vi "DSG Generate Waveform.vi"(6 "hardware commands sync queue":T2, 7 "measurement configuration":T1={"Input channel"=0, "Full scale range"=10.0, "Analog source resource name"="", "Frequency"=1000.0, "Amplitude"=-1.0, "Digital capture resource name"="", "Digital capture sample rate"=800000.0, "Digital capture samples"=800000}, 8 "error in":errorcluster, 10 "DAQmx product name":string, 11 "DSG task in":refnum<k21>) -> (0 "error out":errorcluster, 3 "DSG task out":refnum<k21>)   [LabVIEW 2021, in "AC_ADC.lvlib"]
uses:
  AC_ADC.lvlib
  shared/subVIs/controls/HW Sync Commands Queue Ref.ctl
  shared/subVIs/controls/HW Sync Commands.ctl
  Measurement Configuration.ctl
  <vilib>/addons/_NISVFA/_Generation/Signal Generation/SV Signal/sv_System Timing Model.ctl
  <vilib>/DAQmx/write.llb/DAQmx Write (Analog 1D Wfm NChan NSamp).vi
  <vilib>/addons/_NISVFA/_Generation/Signal Generation/SV Sinusoid/SV Sinusoid.lvclass
  C:/Program Files/National Instruments/LabVIEW 2021/vi.lib/addons/_NISVFA/_Generation/Signal Generation/SV Signal/SV Signal.lvclass
  <vilib>/addons/_NISVFA/_Generation/Signal Generation/SV Sinusoid/Configure Sine.vi
  <vilib>/addons/_NISVFA/_Generation/Signal Generation/SV Signal/Write Sample Rate.vi
  <vilib>/addons/_NISVFA/_Generation/Signal Generation/SV Signal/Write System Timing Model.vi
  <vilib>/addons/_NISVFA/_Generation/Signal Generation/SV Signal/Write Ramp Parameters.vi
  <vilib>/DAQmx/miscellaneous.llb/DAQmx Fill In Error Info.vi
  <resource>/objmgr/daqmx.rc
  <vilib>/addons/_NISVFA/_Generation/Signal Generation/SV Signal/SV Signal.lvclass
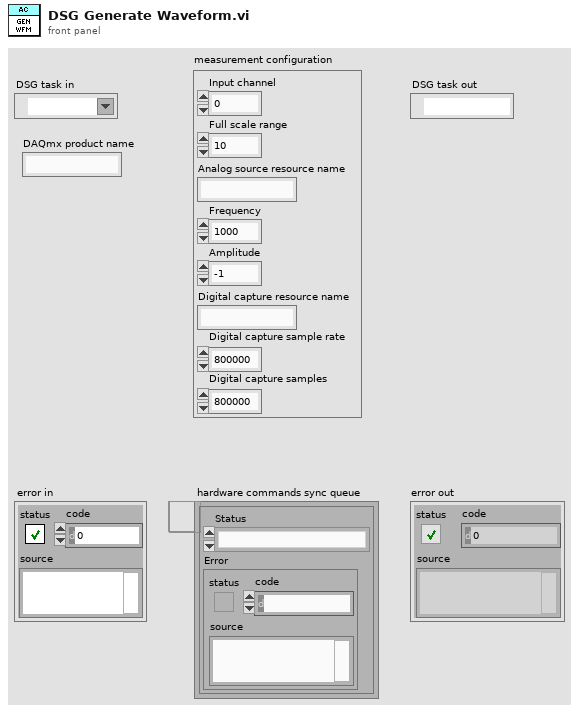
[diagram p1: front panel]
types:
  T1 = typedef "AC_ADC.lvlib/Measurement Configuration.ctl" = cluster{"Input channel":i32, "Full scale range":dbl, "Analog source resource name":string, "Frequency":dbl, "Amplitude":dbl, "Digital capture resource name":string, "Digital capture sample rate":dbl, "Digital capture samples":u32}
  T2 = typedef "HW Sync Commands Queue Ref.ctl" = refnum<queue>
  T3 = enum16{"NoAction", "GenerationStarted", "AcquisitionCompleted", "GenerationErrored"}
  T4 = cluster{"profile":enum16{"Linear", "Half cosine"}, "durations [s]":cluster{"ramp-up":dbl, "transition":dbl, "ramp-down":dbl}}
  T5 = typedef "HW Sync Commands.ctl" = enum16{"NoAction", "GenerationStarted", "AcquisitionCompleted", "GenerationErrored"}
  T6 = cluster{"element":enum16{"NoAction", "GenerationStarted", "AcquisitionCompleted", "GenerationErrored"}, "error out":errorcluster}
  T7 = typedef "SV Signal.lvclass/sv_System Timing Model.ctl" = i64
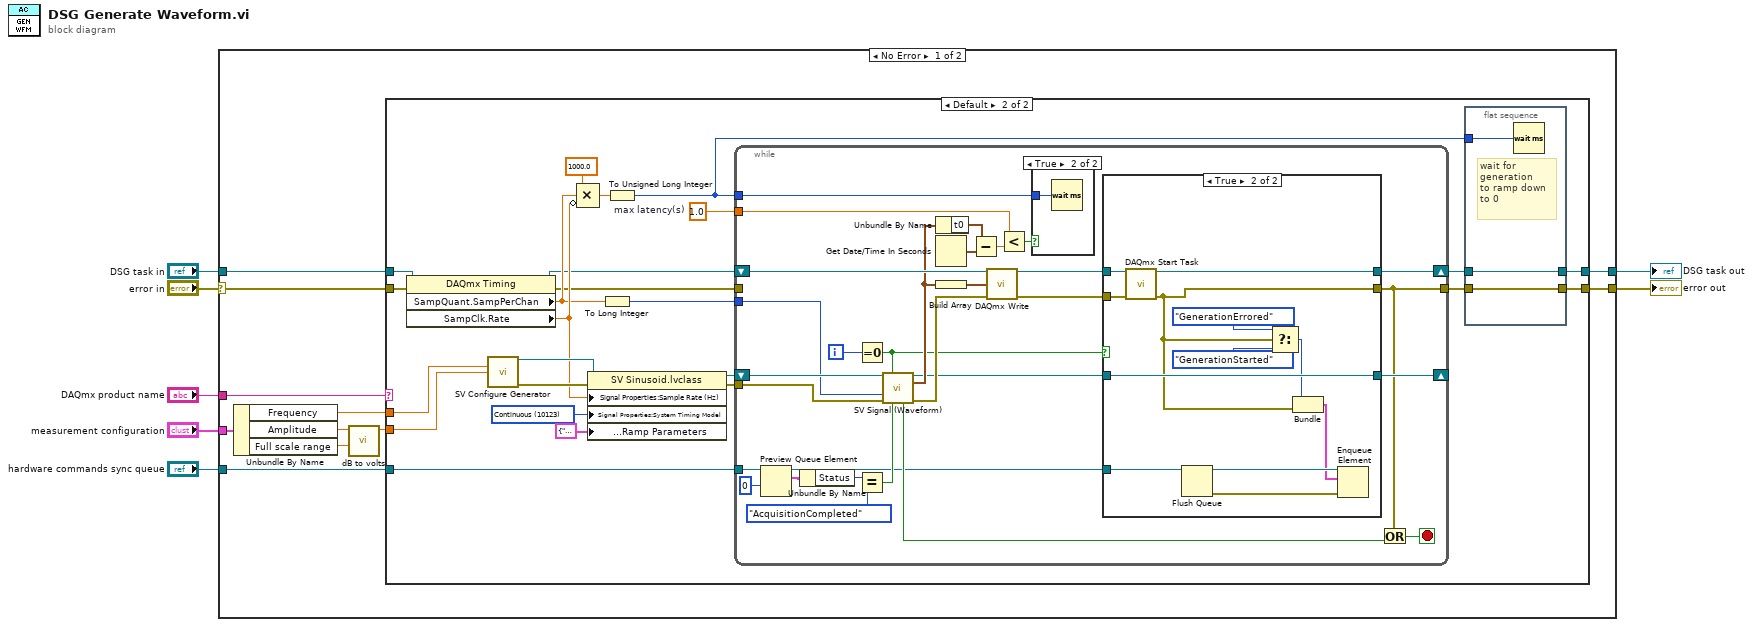
[diagram p0: block diagram]
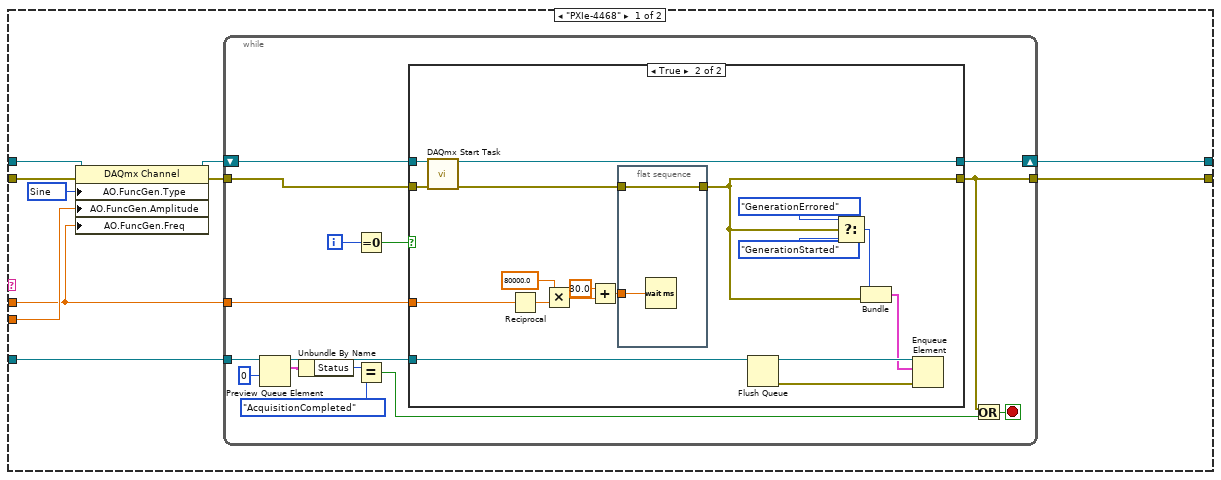
[diagram p2: hidden frame]
diagram:
  n1 = case shown="No Error" "error in" {
    selector: "error in" -> [w18 w140]
    tunnel: [w17 w139] -> w6
    tunnel: [w16 w140] -> w5
    tunnel: "DSG task in" -> [w10 w139]
    tunnel: "hardware commands sync queue" -> [w15 _]
    tunnel: "measurement configuration" -> [w14 _]
    tunnel: "DAQmx product name" -> [w9 _]
    frame No Error {
      n2 = Unbundle By Name(w14) -> ("Frequency"=w12:dbl, "Amplitude"=w13:dbl, "Full scale range"=w8:dbl)
      n3 = call "dB to volts.vi"("Full scale range"=w8, "Voltage(dB)"=w13) -> ("Voltage(volts)"=w11:dbl)  [unwired: 9 in]
      n4 = case shown="Default" w9 {
        tunnel: w18 -> [w22 w89]
        tunnel: w10 -> [w24 w85]
        tunnel: [w27 w73] -> w17
        tunnel: [w26 w72] -> w16
        tunnel: w15 -> [w28 w70]
        tunnel: w12 -> [w19 w68]
        tunnel: w11 -> [w20 w67]
        frame "PXIe-4468" {
          w21 = 14751 items=["Sine"=14751, "Triangle"=14752, "Square"=14753, "Sawtooth"=14754] ("AO.FuncGen.Type")
          n5 = property class="DAQmx Channel"(reference=w24, error in=w22, "AO.FuncGen.Type"=w21, "AO.FuncGen.Amplitude"=w20, "AO.FuncGen.Freq"=w19) -> (reference out=w25:refnum<k21>, error out=w23:errorcluster)
          n6 = while {
            tunnel: w23 -> [w42]
            shift-right: [w36] -> w27
            shift-left: w25 -> [w41]
            tunnel: [w29] -> w26
            tunnel: w28 -> [w33]
            tunnel: w19 -> [w30]
            i -> [w43]
            stop <- w40 stop-if-true
            n7 = Preview Queue Element(queue=w33, timeout in ms (-1)=0) -> (queue out=w37:T2, element=w35:cluster{"Status":T5, "Error":errorcluster})  [unwired: 1 in, 2 out]
            n8 = Unbundle By Name(w35) -> ("Status"=w34:T5)
            n9 = Equal To 0?(x=w43) -> (x = 0?=w32:bool)
            n10 = Equal?(x=w34, y=T3."AcquisitionCompleted") -> (x = y?=w31:bool)
            n11 = case shown="True" w32 {
              tunnel: w37 -> [_ w63]
              tunnel: w41 -> [w45 w61]
              tunnel: [w45 w47] -> w36
              tunnel: w42 -> [w44 w60]
              tunnel: [w44 w49] -> w29
              tunnel: w30 -> [_ w46]
              frame False {
              }
              frame True {
                n12 = call <vilib>:"DAQmx Start Task.vi"("task/channels in"=w61, "error in"=w60) -> ("task out"=w47:refnum<k21>, "error out"=w50:errorcluster)  [unwired: 12 in]
                n13 = Reciprocal(x=w46) -> (1/x=w51:dbl)
                n14 = Multiply(x=80000.0, y=w51) -> (x*y=w53:dbl)
                n15 = Add(x=30.0, y=w53) -> (x+y=w48:dbl)
                n16 = flat-sequence {
                  tunnel: w50 -> [w65]
                  tunnel: [w65] -> w49
                  tunnel: w48 -> [w64]
                  frame #0 {
                    n17 = Wait (ms)(milliseconds to wait=w64) -> ()  [unwired: 1 out]
                  }
                }
                n18 = Flush Queue(queue=w63) -> (queue out=w62:T2, error out=w59:errorcluster)  [unwired: 1 in, 1 out]
                n19 = Select(t=T3."GenerationErrored" ("element"), s=w49, f=T3."GenerationStarted" ("element")) -> (s? t:f=w56:T3)
                n20 = Bundle("element"=w56, "error out"=w49) -> (w55:T6)  [unwired: 1 in]
                n21 = Enqueue Element(queue=w62, element=w55, error in (no error)=w59) -> ()  [unwired: 1 in, 3 out]
              }
            }
            n22 = Or(x=w29, y=w31) -> (x .or. y?=w40:bool)
          }
        }
        frame Default {
          w78 = 1.0  # max latency(s)
          w86 = T7 10123 items=["Finite"=10178, "-"=-1, "Continuous"=10123, "-"=-2, "Settled"=110123, "Averaged"=210123, "Discrete Sweep"=310123, "Continuous Sweep"=410123] ("System Timing Model")
          n23 = property class="DAQmx Timing"(reference=w85, error in=w89) -> (reference out=w79:refnum<k21>, error out=w66:errorcluster, "SampQuant.SampPerChan"=w81:dbl, "SampClk.Rate"=w84:dbl)
          n24 = call-poly <vilib>:"SV Configure Generator.vi"("frequency (Hz)"=w68, "amplitude"=w67) -> ("signal configuration"=w87:refnum<class "SV Sinusoid.lvclass">, "error out"=w88:errorcluster)  [unwired: 12 in]
          n25 = Compound Arithmetic op=MULTIPLY(1000.0 ("value"), w81, invert w84) -> (w77:dbl)
          n26 = property class="SV Sinusoid.lvclass"(reference=w87, error in=w88, "Signal Properties:Sample Rate (Hz)"=w84, "Signal Properties:System Timing Model"=w86, "Signal Properties:Ramps:Ramp Parameters"=T4 {"profile"=enum."Linear", "durations [s]"={"ramp-up"=0.0, "transition"=0.0, "ramp-down"=0.01}} ("Ramp Parameters:All Elements")) -> (reference out=w83:refnum<class "SV Sinusoid.lvclass">, error out=w82:errorcluster)
          n27 = To Long Integer(number=w81) -> (32bit integer=w80:i32)
          n28 = To Unsigned Long Integer(number=w77) -> (unsigned 32bit integer=w71:u32)
          n29 = while {
            shift-right: [w96] -> _
            shift-left: w83 -> [w122]
            tunnel: w82 -> [w119]
            tunnel: w80 -> [w120]
            shift-right: [w99] -> w74
            shift-left: w79 -> [w118]
            tunnel: [w93] -> w75
            tunnel: w78 -> [w109]
            tunnel: w71 -> [w107]
            tunnel: w70 -> [w106]
            tunnel: w66 -> [_]
            i -> [w121]
            stop <- w114 stop-if-true
            n30 = Preview Queue Element(queue=w106, timeout in ms (-1)=0) -> (queue out=w102:T2, element=w95:cluster{"Status":T5, "Error":errorcluster})  [unwired: 1 in, 2 out]
            n31 = Unbundle By Name(w95) -> ("Status"=w94:T5)
            n32 = Equal To 0?(x=w121) -> (x = 0?=w101:bool)
            n33 = Equal?(x=w94, y=HW_Sync_Commands."AcquisitionCompleted") -> (x = y?=w103:bool)
            n34 = call-dynamic "SV Signal (Waveform).vi"("signal configuration"=w122, "reset"=w101, "samples"=w120, "error in (no error)"=w119, "stop"=w103) -> ("signal configuration"=w97:refnum<class "SV Sinusoid.lvclass">, "output waveform"=w113:waveform(dbl), "done"=w115:bool, "error out"=w116:errorcluster)  [unwired: 5 in, 2 out]
            n35 = Unbundle By Name(w113) -> ("t0"=w112:timestamp)
            n36 = Get Date/Time In Seconds() -> (seconds since 1Jan1904=w111:timestamp)
            n37 = Build Array(w113) -> (w117:waveform(dbl)[])
            n38 = Subtract(x=w112, y=w111) -> (x-y=w110:dbl)
            n39 = call-poly <vilib>:"DAQmx Write.vi"("task/channels in"=w118, "data"=w117, "error in"=w116) -> ("task out"=w100:refnum<k21>, "error out"=w98:errorcluster)  [unwired: 10 in, 1 out]
            n40 = Less?(x=w109, y=w110) -> (x < y?=w108:bool)
            n41 = case shown="True" w108 {
              tunnel: w107 -> [_ w138]
              frame False {
              }
              frame True {
                n42 = Wait (ms)(milliseconds to wait=w138) -> ()  [unwired: 1 out]
              }
            }
            n43 = case shown="True" w101 {
              tunnel: w102 -> [_ w137]
              tunnel: w100 -> [w125 w135]
              tunnel: [w125 w134] -> w99
              tunnel: w98 -> [w124 w133]
              tunnel: [w124 w127] -> w93
              tunnel: w97 -> [w123 w129]
              tunnel: [w123 w129] -> w96
              frame False {
              }
              frame True {
                n44 = call <vilib>:"DAQmx Start Task.vi"("task/channels in"=w135, "error in"=w133) -> ("task out"=w134:refnum<k21>, "error out"=w127:errorcluster)  [unwired: 12 in]
                n45 = Flush Queue(queue=w137) -> (queue out=w136:T2, error out=w132:errorcluster)  [unwired: 1 in, 1 out]
                n46 = Select(t=HW_Sync_Commands."GenerationErrored" ("element"), s=w127, f=HW_Sync_Commands."GenerationStarted" ("element")) -> (s? t:f=w128:T5)
                n47 = Bundle("element"=w128, "error out"=w127) -> (w126:cluster{"element":T5, "error out":errorcluster})  [unwired: 1 in]
                n48 = Enqueue Element(queue=w136, element=w126, error in (no error)=w132) -> ()  [unwired: 1 in, 3 out]
              }
            }
            n49 = Or(x=w93, y=w115) -> (x .or. y?=w114:bool)
          }
          n50 = flat-sequence {
            tunnel: w75 -> [w91]
            tunnel: w74 -> [w92]
            tunnel: [w92] -> w73
            tunnel: [w91] -> w72
            tunnel: w71 -> [w90]
            frame #0 {
              # "wait for\ngeneration\nto ramp down\nto 0"
              n51 = Wait (ms)(milliseconds to wait=w90) -> ()  [unwired: 1 out]
            }
          }
        }
      }
    }
    frame Error {
    }
  }
  "DSG task out" <- w6
  "error out" <- w5
